vi "log file header.vi"(9 "method":T1={"integration time (s)"=0.5, "shortest wavelength"=190.0, "longest wavelength"=820.0, "sample interval (s)"=2.0, "delay (s)"=0.5} {"delay (s)" min=0 max=25.5 step=0.1 format="%.1f"; "sample interval (s)" min=1.1 max=99999.9 step=0.1 format="%.1f"; "longest wavelength" min=190 max=820 step=1; "shortest wavelength" min=190 max=820 step=1; "integration time (s)" min=0.1 max=25.5 step=0.1 format="%.1f"}, 10 "mixture cluster":T2 {"H array" format="%.2f"}, 11 "file path":refnum<file>) -> ()   [LabVIEW 2015]
uses:
  mixture cluster.ctl
  Continuous settings.ctl
panel:
  out "file path out":refnum<file>
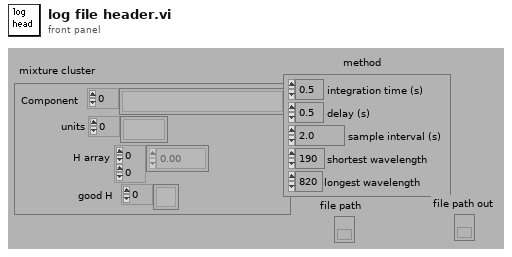
[diagram p1: front panel]
types:
  T1 = typedef "Continuous settings.ctl" = cluster{"integration time (s)":sgl, "shortest wavelength":sgl, "longest wavelength":sgl, "sample interval (s)":dbl, "delay (s)":sgl}
  T2 = typedef "mixture cluster.ctl" = cluster{"Component":string[], "units":string[], "H array":dbl[][], "good H":bool[]}
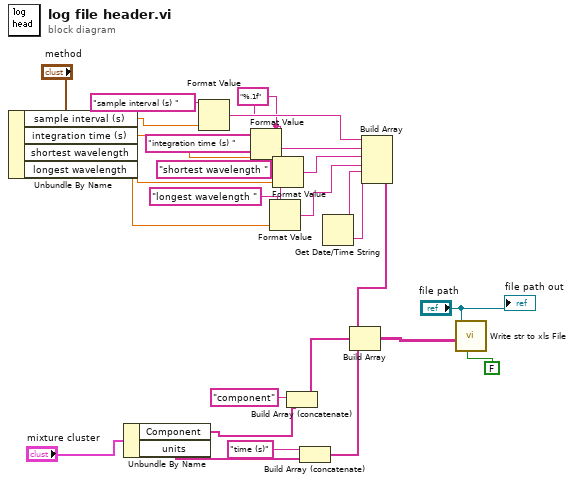
[diagram p0: block diagram]
diagram:
  w11 = "%.1f"
  n1 = Unbundle By Name("method") -> ("sample interval (s)"=w22:dbl, "integration time (s)"=w25:sgl, "shortest wavelength"=w20:sgl, "longest wavelength"=w13:sgl)
  n2 = Unbundle By Name("mixture cluster") -> ("Component"=w7:string[], "units"=w6:string[])
  n3 = Format Value(string ("")="sample interval (s) ", format string=w11, value (0)=w22) -> (output string=w24:string)
  n4 = Format Value(string ("")="integration time (s) ", format string=w11, value (0)=w25) -> (output string=w27:string)
  n5 = Format Value(string ("")="longest wavelength ", format string=w11, value (0)=w13) -> (output string=w10:string)
  n6 = Format Value(string ("")="shortest wavelength ", format string=w11, value (0)=w20) -> (output string=w19:string)
  n7 = Build Array (concatenate)("component", w7) -> (w4:string[])
  n8 = Build Array (concatenate)("time (s)", w6) -> (w3:string[])
  n9 = Get Date/Time String() -> (date string=w14:string, time string=w18:string)  [unwired: 3 in]
  n10 = Build Array(w24, w27, w19, w10, w14, w18) -> (w5:string[])
  n11 = Build Array(w5, w4, w3) -> (w2:string[][])
  n12 = call "Write str to xls File.vi"("transpose? (no:F)"=FALSE, "2D data"=w2, "refnum"="file path") -> ()  [unwired: 7 in, 2 out]
  "file path out" <- "file path"
